vi "read_counter.vi"() -> ()   [LabVIEW 2011]
panel:
  out "TCP Error":errorcluster
  out "Deque error":errorcluster
  out "DataSocket error":errorcluster
  out "# Sent Data":u64
  out "Data from people counter":string
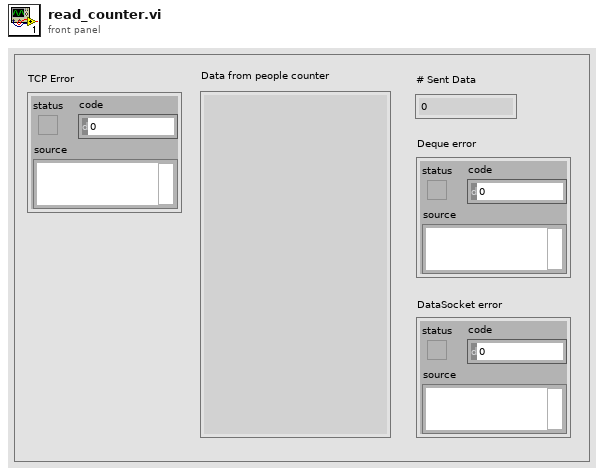
[diagram p1: front panel]
types:
  T1 = enum16{"Read", "Write", "ReadWrite", "BufferedRead", "BufferedReadWrite"}
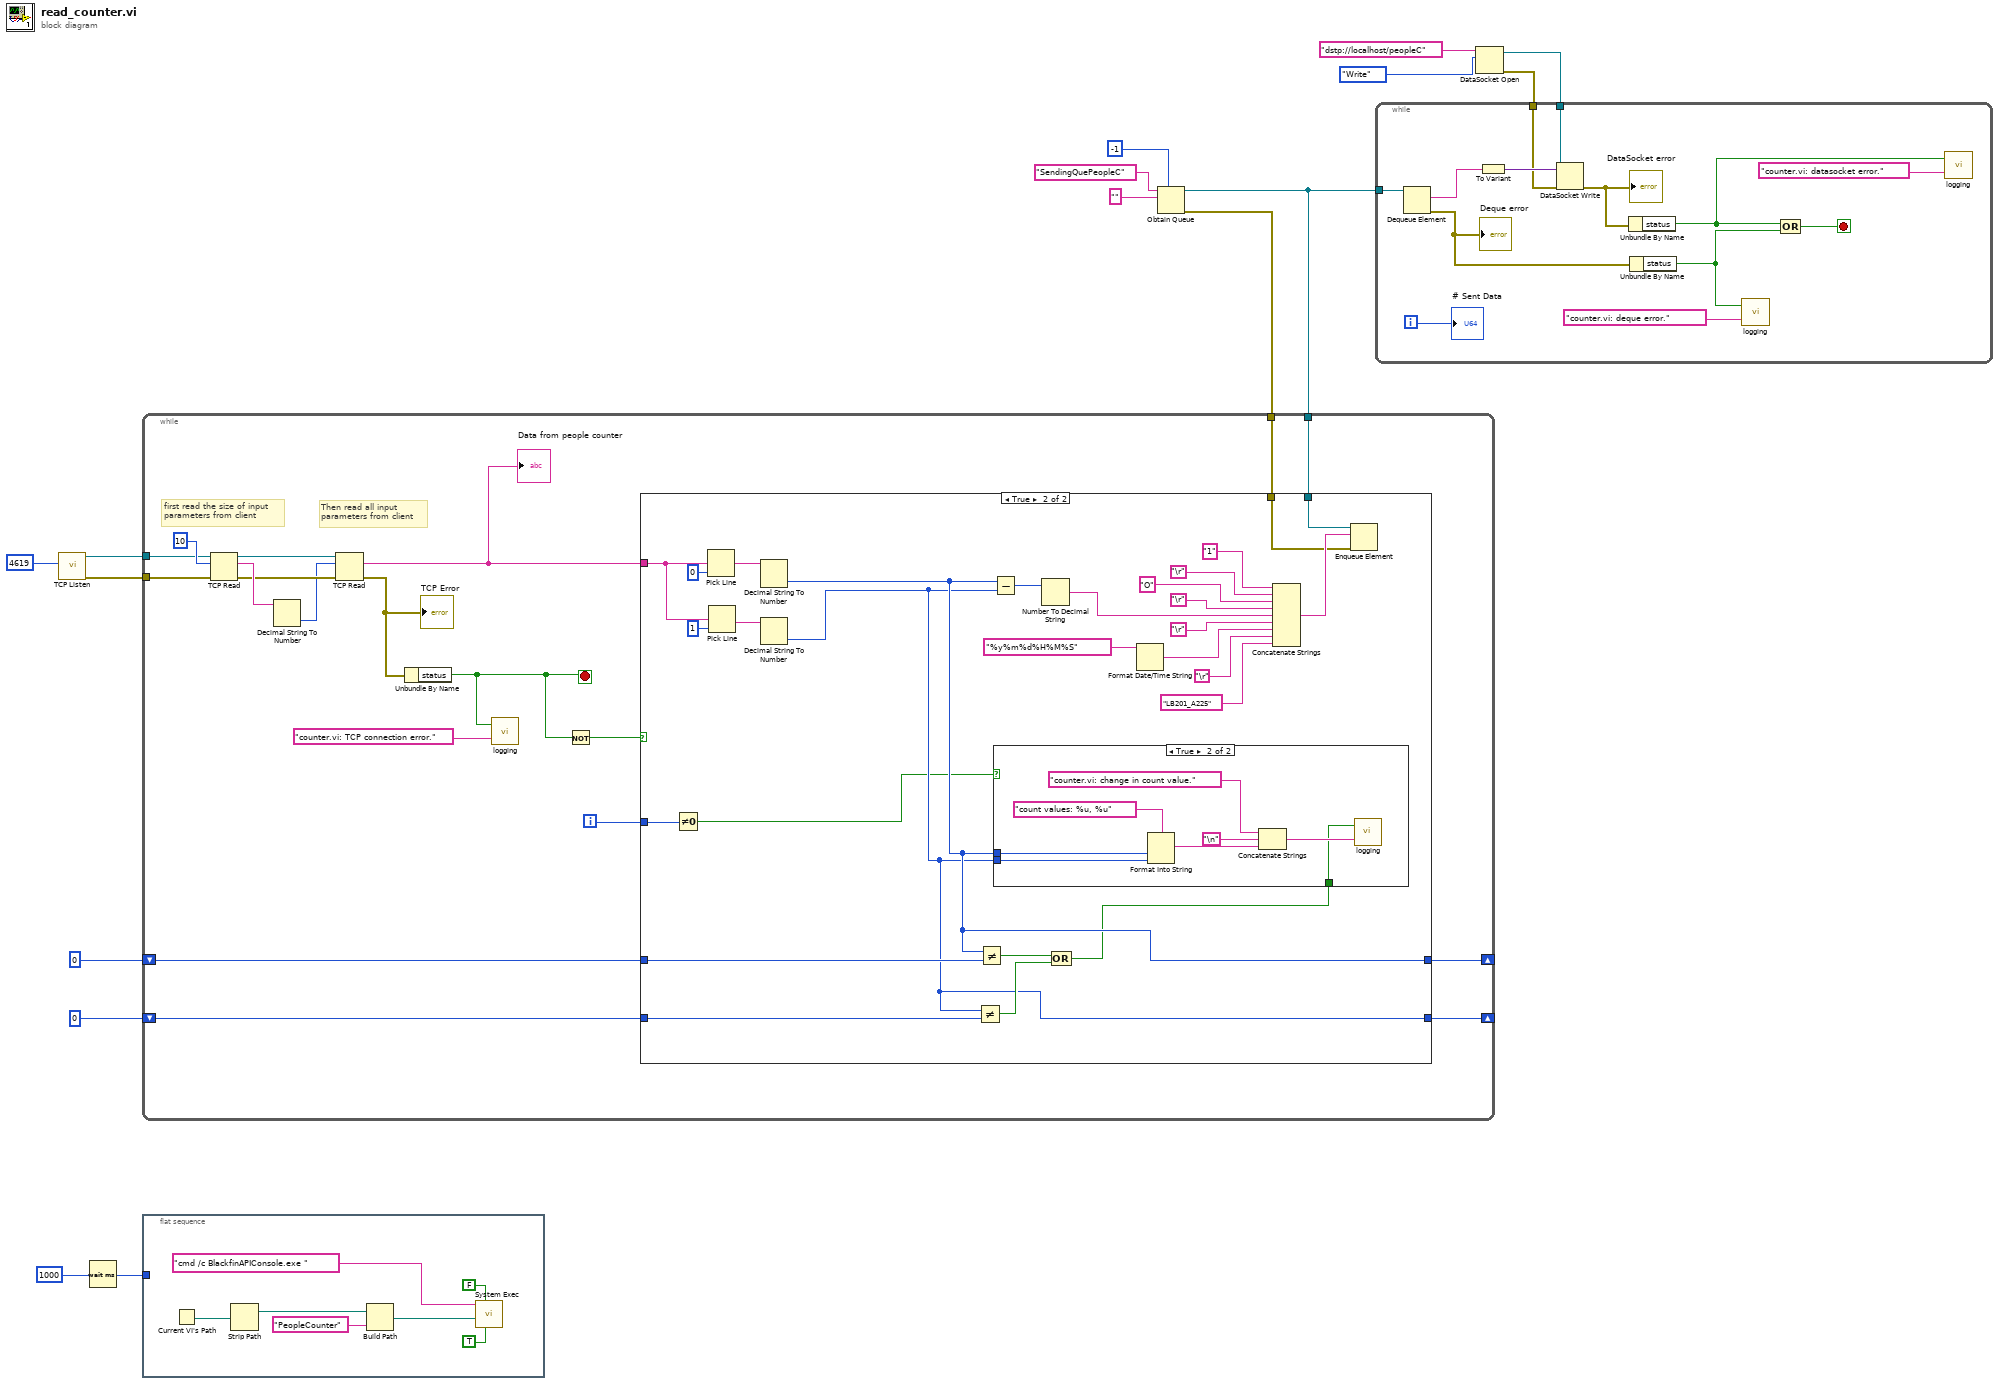
[diagram p0: block diagram]
diagram:
  n1 = call <vilib>:"TCP Listen.vi"("port"=u16 4619) -> ("error out"=w15:errorcluster, "connection ID"=w16:refnum<k5>)  [unwired: 6 in, 3 out]
  n2 = Wait (ms)(milliseconds to wait=u32 1000) -> (millisecond timer value=w3:u32)
  n3 = flat-sequence {
    tunnel: w3 -> [_]
    frame #0 {
      n4 = Current VI's Path() -> (path=w23:path)
      n5 = Strip Path(path=w23) -> (stripped path=w19:path)  [unwired: 1 out]
      n6 = Build Path(base path=w19, name or relative path="PeopleCounter") -> (appended path=w17:path)
      n7 = call <vilib>:"System Exec.vi"("run minimized? (F)"=TRUE, "wait until completion? (T)"=FALSE, "working directory"=w17, "command line"="cmd /c BlackfinAPIConsole.exe ") -> ()  [unwired: 4 in, 4 out]
    }
  }
  n8 = Obtain Queue(max queue size (-1, unlimited)=-1, name (unnamed)="SendingQuePeopleC", element data type="") -> (queue out=w8:refnum<queue>, error out=w6:errorcluster)  [unwired: 2 in, 1 out]
  n9 = while {
    tunnel: w16 -> [w37]
    tunnel: w15 -> [w36]
    tunnel: w8 -> [w35]
    tunnel: w6 -> [w34]
    shift-right: [w26] -> _
    shift-left: 0 -> [w33]
    shift-right: [w25] -> _
    shift-left: 0 -> [w32]
    i -> [w24]
    stop <- w27 stop-if-true
    # "Then read all input \nparameters from client"
    # "first read the size of input \nparameters from client"
    n10 = TCP Read(connection ID=w37, bytes to read=10, error in (no error)=w36) -> (connection ID out=w40:refnum<k5>, data out=w41:string, error out=w39:errorcluster)  [unwired: 2 in]
    n11 = Decimal String To Number(string=w41) -> (number=w38:i32)  [unwired: 2 in, 1 out]
    n12 = TCP Read(connection ID=w40, bytes to read=w38, error in (no error)=w39) -> (data out=w31:string, error out=w29:errorcluster)  [unwired: 2 in, 1 out]
    "Data from people counter" <- w31
    "TCP Error" <- w29
    n13 = Unbundle By Name(w29) -> ("status"=w27:bool)
    n14 = call "logging.vi"("data"="counter.vi: TCP connection error.", "Boolean"=w27) -> ()  [unwired: 1 in]
    n15 = Not(x=w27) -> (.not. x?=w28:bool)
    n16 = case shown="True" w28 {
      tunnel: w35 -> [_ w62]
      tunnel: w34 -> [_ w61]
      tunnel: w33 -> [w44 w58]
      tunnel: w32 -> [w43 w57]
      tunnel: w31 -> [_ w51]
      tunnel: [w44 w49] -> w26
      tunnel: [w43 w48] -> w25
      tunnel: w24 -> [_ w46]
      frame False {
      }
      frame True {
        n17 = Not Equal To 0?(x=w46) -> (x != 0?=w45:bool)
        n18 = Pick Line(multi-line string=w51, line index=0) -> (output string=w53:string)  [unwired: 1 in]
        n19 = Pick Line(multi-line string=w51, line index=1) -> (output string=w50:string)  [unwired: 1 in]
        n20 = Decimal String To Number(string=w53) -> (number=w49:i32)  [unwired: 2 in, 1 out]
        n21 = Decimal String To Number(string=w50) -> (number=w48:i32)  [unwired: 2 in, 1 out]
        n22 = Not Equal?(x=w48, y=w57) -> (x != y?=w55:bool)
        n23 = Not Equal?(x=w49, y=w58) -> (x != y?=w56:bool)
        n24 = Subtract(x=w49, y=w48) -> (x-y=w65:i32)
        n25 = Number To Decimal String(number=w65) -> (decimal integer string=w64:string)  [unwired: 1 in]
        n26 = Compound Arithmetic op=OR(w56, w55) -> (w47:bool)
        n27 = case shown="True" w45 {
          tunnel: w49 -> [_ w75]
          tunnel: w48 -> [_ w74]
          tunnel: w47 -> [_ w73]
          frame False {
          }
          frame True {
            n28 = Format Into String(format string="count values: %u, %u", w75, w74) -> (resulting string=w76:string)  [unwired: 2 in, 1 out]
            n29 = Concatenate Strings("counter.vi: change in count value.", "\n", w76) -> (w78:string)
            n30 = call "logging.vi"("data"=w78, "Boolean"=w73) -> ()  [unwired: 1 in]
          }
        }
        n31 = Format Date/Time String(time format string (%c)="%y%m%d%H%M%S") -> (date/time string=w59:string)  [unwired: 2 in]
        n32 = Concatenate Strings("1" ("string"), "\r", "O" ("string"), "\r", w64, "\r", w59, "\r", "LB201_A225") -> (w63:string)
        n33 = Enqueue Element(queue=w62, element=w63, error in (no error)=w61) -> ()  [unwired: 1 in, 3 out]
      }
    }
  }
  n34 = DataSocket Open(10:T1."Write" ("mode"), 11:"dstp://localhost/peopleC" ("URL 3")) -> (0:w14:errorcluster, 3:w13:refnum<k13>)  [unwired: 2 in]
  n35 = while {
    tunnel: w8 -> [w93]
    tunnel: w13 -> [w92]
    tunnel: w14 -> [w87]
    i -> [w85]
    stop <- w86 stop-if-true
    n36 = Dequeue Element(queue=w93) -> (element=w90:string, error out=w89:errorcluster)  [unwired: 2 in, 2 out]
    "Deque error" <- w89
    n37 = To Variant(anything=w90) -> (Variant=w91:variant)
    n38 = DataSocket Write(8:w87, 10:w91, 11:w92) -> (0:w88:errorcluster)  [unwired: 3 out]
    "DataSocket error" <- w88
    n39 = Unbundle By Name(w88) -> ("status"=w81:bool)
    n40 = Unbundle By Name(w89) -> ("status"=w83:bool)
    n41 = call "logging.vi"("data"="counter.vi: deque error.", "Boolean"=w83) -> ()  [unwired: 1 in]
    n42 = Compound Arithmetic op=OR(w81, w83) -> (w86:bool)
    n43 = call "logging.vi"("data"="counter.vi: datasocket error.", "Boolean"=w81) -> ()  [unwired: 1 in]
    "# Sent Data" <- w85
  }
